vi "CrossC2.vi"(6 "Synchronization":enum16{"Start", "Wait"}(ring), 7 "Description":string, 8 "Command Info In":T1, 10 "Duration (s)":dbl, 11 "Setpoint":dbl) -> (0 "Command Info Out":T1)   [LabVIEW 2015]
uses:
  <vilib>/Rock Robotics/WPI/Framework/Command Status Info.ctl
  <vilib>/Rock Robotics/WPI/Framework/Completion Status.ctl
  <vilib>/Rock Robotics/WPI/Framework/Completion Notifier.ctl
  Implementation/AutoTask Setpoints.ctl
  Implementation/AutoTask Operations.ctl
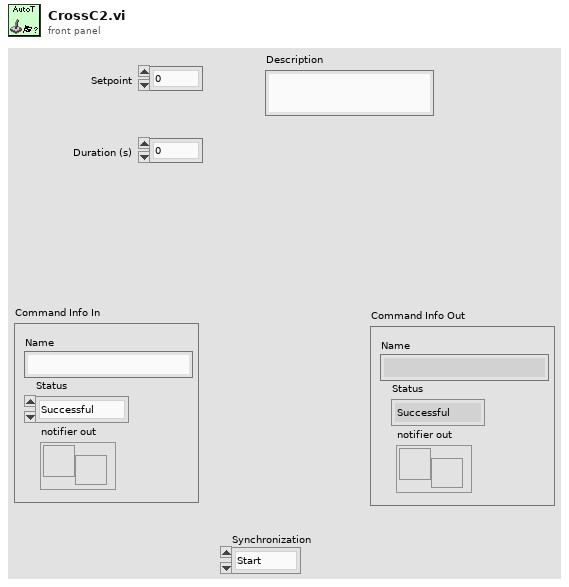
[diagram p1: front panel]
types:
  T1 = typedef "Command Status Info.ctl" = cluster{"Name":string, "Status":T2, "notifier out":T3}
  T2 = typedef "Completion Status.ctl" = enum16{"Successful", "Aborted", "Incomplete"}
  T3 = typedef "Completion Notifier.ctl" = refnum<notifier>
  T4 = typedef "AutoTask Setpoints.ctl" = cluster{"Operation":T5, "Setpoint":dbl, "Duration":dbl, "Speed":dbl, "Angle":dbl, "VDeadband":dbl, "Deadband":dbl, "DriveSpeed":dbl}
  T5 = typedef "AutoTask Operations.ctl" = enum16{"Reserve", "Read Current", "Immediate", "DriveDistance", "AutoShoot", "FaceForward", "AutoAlign", "AutoTurn", "DriveToLine", "CrossLB", "CrossD2", "CrossD1", "CrossC2", "CrossC1", "CrossB2", "CrossB1", "CrossA2", "CrossA1"}
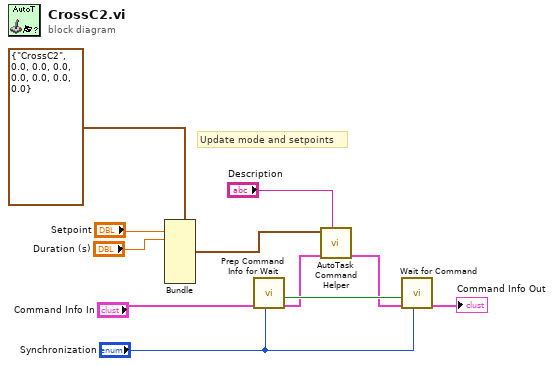
[diagram p0: block diagram]
diagram:
  # "Update mode and setpoints"
  n1 = Bundle(cluster=T4 {"Operation"=enum."CrossC2", "Setpoint"=0.0, "Duration"=0.0, "Speed"=0.0, "Angle"=0.0, "VDeadband"=0.0, "Deadband"=0.0, "DriveSpeed"=0.0} ("SubSystem Data"), "Setpoint"="Setpoint", "Duration"="Duration (s)") -> (w3:T4)  [unwired: 6 in]
  n2 = call <vilib>:"Prep Command Info for Wait.vi"("Synchronication"="Synchronization", "Command Info"="Command Info In") -> ("Command Info"=w7:T1, "Allocated"=w8:bool)  [unwired: 8 in]
  n3 = call "AutoTask Command Helper.vi"("Description"="Description", "Command Info In"=w7, "SubSystem Data"=w3) -> ("Command Info Out"=w4:T1)  [unwired: 7 in, 1 out]
  n4 = call <vilib>:"Wait for Command.vi"("Synchronication"="Synchronization", "Command Info in"=w4, "Allocated"=w8) -> ("Command Info out"=→"Command Info Out":T1)  [unwired: 8 in]
